vi "Get Created Events.vi"(11 "Queue Mailbox in":refnum<class "Queue Mailbox.lvclass">) -> (2 "Created Events":map{string, refnum<data-value>}(c390))   [LabVIEW 2021, in "jettl.lvlib" / "Queue Mailbox.lvlib" / "Queue Mailbox.lvclass"]
uses:
  Queue Mailbox.lvclass
  Msg Strategy/Msg Strategy.lvclass
  Queue Mailbox.lvclass/Queue Mailbox.ctl
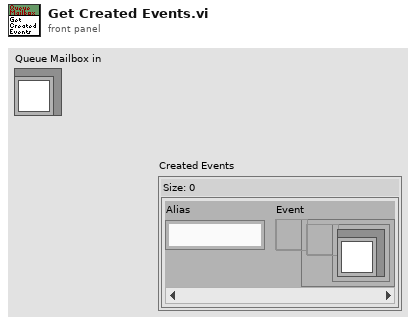
[diagram p1: front panel]
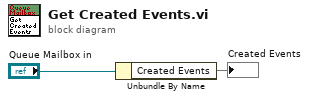
[diagram p0: block diagram]
diagram:
  n1 = Unbundle By Name("Queue Mailbox in") -> ("Created Events"=→"Created Events":map{string, refnum<data-value>})
